vi "Set Harmonics.vi"(6 "PLL source (0: V1)":u16(ring) items=["V1", "A1", "V2", "A2", "V3", "A3"], 8 "error in (no error)":errorcluster, 9 "Element (1: Element 1)":u16(ring)=1 items=["", "Element1", "Element2", "Element3"], 10 "Harmonic Mode (F: OFF)":bool, 11 "Universal Power Meter in":refnum<class "Universal Power Meter.lvclass">) -> (0 "error out":errorcluster, 2 "Power Meter Visa":refnum<visa-resource-name>, 3 "Universal Power Meter out":refnum<class "Universal Power Meter.lvclass">)   [LabVIEW 2012, in "Universal Power Meter.lvlib" / "Universal Power Meter.lvclass"]
uses:
  Universal Power Meter.lvclass
  Universal Power Meter.lvclass/Universal Power Meter.ctl
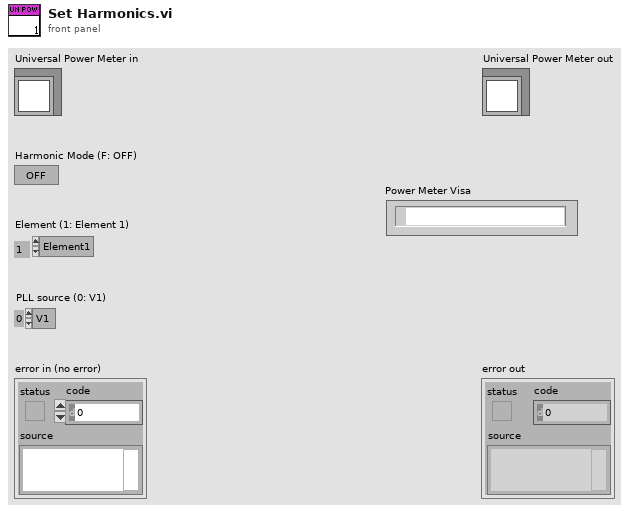
[diagram p1: front panel]
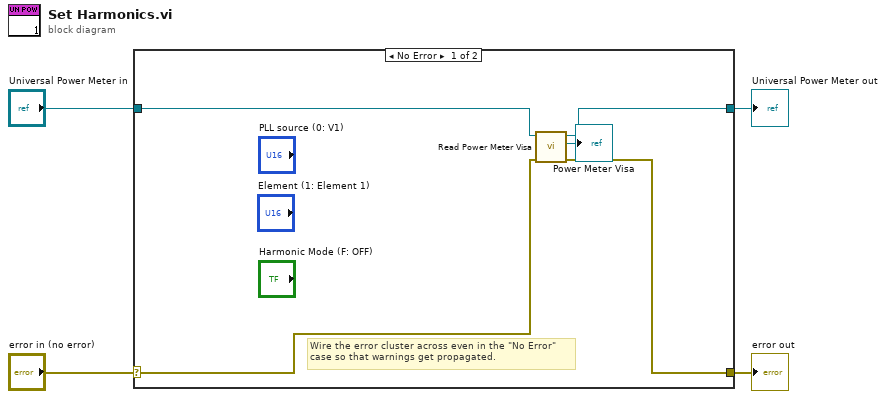
[diagram p0: block diagram]
diagram:
  n1 = case shown="No Error" "error in (no error)" {
    selector: "error in (no error)" -> [w7 w11]
    tunnel: [w6 w11] -> w3
    tunnel: [w8 w10] -> w1
    tunnel: "Universal Power Meter in" -> [w9 w10]
    frame No Error {
      # "Wire the error cluster across even in the \"No Error\"\ncase so that warnings get propagated."
      n2 = call "Read Power Meter Visa.vi"("error in (no error)"=w7, "Universal Power Meter in"=w9) -> ("error out"=w6:errorcluster, "Power Meter Visa"=→"Power Meter Visa":refnum<visa-resource-name>, "Universal Power Meter out"=w8:refnum<class "Universal Power Meter.lvclass">)  [unwired: 7 in]
    }
    frame Error {
    }
  }
  "error out" <- w3
  "Universal Power Meter out" <- w1
